vi "Read ClkHandle.vi"(8 "error in (no error)":errorcluster, 11 "SensorBase in":refnum<class "SensorBase.lvclass">) -> (0 "error out":errorcluster, 2 "ClkHandle":variant, 3 "SensorBase out":refnum<class "SensorBase.lvclass">)   [LabVIEW 2018, in "SensorPlugins.lvlib" / "SensorBase.lvclass"]
uses:
  SensorBase.lvclass
  SensorBase.lvclass/SensorBase.ctl
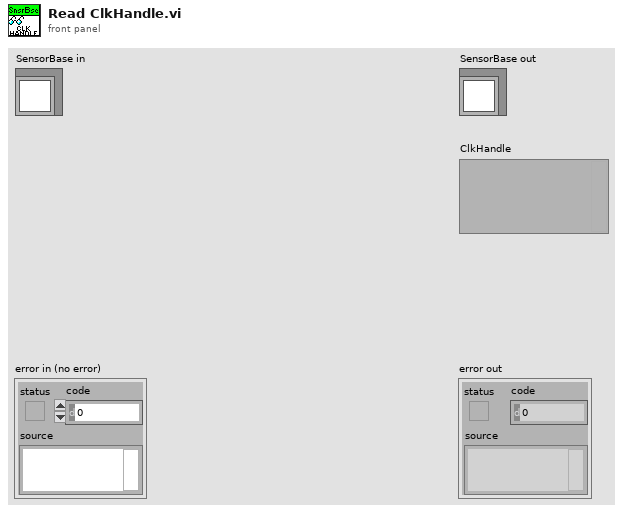
[diagram p1: front panel]
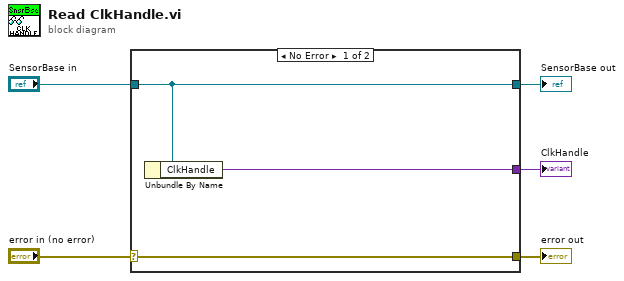
[diagram p0: block diagram]
diagram:
  n1 = case shown="No Error" "error in (no error)" {
    selector: "error in (no error)" -> [w8 w9]
    tunnel: [w8 w9] -> w4
    tunnel: [w7 w10] -> w2
    tunnel: "SensorBase in" -> [w7 w10]
    tunnel: [w6 _] -> w1
    frame No Error {
      n2 = Unbundle By Name(w7) -> ("ClkHandle"=w6:variant)
    }
    frame Error {
    }
  }
  "error out" <- w4
  "SensorBase out" <- w2
  "ClkHandle" <- w1
